vi "Xbox Controller.vi"   [LabVIEW 2011]
uses:
  _GlobalVariables&Libraries/ATV Program Global Variables.vi
types:
  T1 = cluster{"X axis":i32, "Y axis":i32, "Z axis":i32, "X axis rotation":i32, "Y axis rotation":i32, "Z axis rotation":i32, "U axis":i32, "V axis":i32}
  T2 = cluster{"button 1":bool, "button 2":bool, "button 3":bool, "button 4":bool, "button 5":bool, "button 6":bool, "button 7":bool, "button 8":bool, "button 9":bool, "button 10":bool, "button 11":bool, "button 12":bool, "button 13":bool, "button 14":bool, "button 15":bool, "button 16":bool, "button 17":bool, "button 18":bool, "button 19":bool, "button 20":bool, "button 21":bool, "button 22":bool, "button 23":bool, "button 24":bool, "button 25":bool, "button 26":bool, "button 27":bool, "button 28":bool, "button 29":bool, "button 30":bool, "button 31":bool, "button 32":bool}
  T3 = cluster{"pov 1":i32, "pov 2":i32, "pov 3":i32, "pov 4":i32}
  T4 = cluster{"End ATV Program":bool, "E-Stop":bool, "Save Logfile":bool, "Logfile Iteration Delay (ms)":u32, "Loop iteration time (ms)":u32, "Logfile Location":path, "Default GPS Navigation Path":path, "Computer":string, "Default GPS Boundary Path":path}
  T5 = cluster{"Drive Value Output String":string, "Steer Value Output String":string, "Button A":bool, "Button B":bool, "Error Out":errorcluster, "Disable XBox Drive & Steer":bool, "Disable XBox Controller":bool, "XBOX Button Trigger Time (ms)":u32, "Button X":bool, "Button Y":bool}
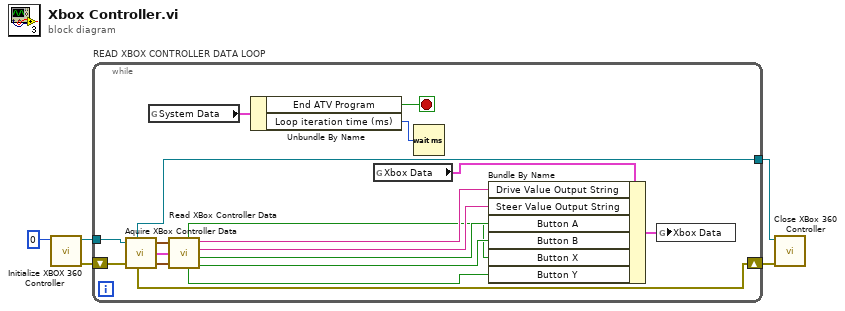
[diagram p0: block diagram]
diagram:
  n1 = call "Initialize XBOX 360 Controller.vi"("XBox Device Index"=0) -> ("Rrror Out"=w3:errorcluster, "Device ID"=w5:refnum<k1>)  [unwired: 8 in, 1 out]
  n2 = while "READ XBOX CONTROLLER DATA LOOP" {
    tunnel: [w20] -> w2
    tunnel: w5 -> [w19]
    shift-right: [w17] -> w1
    shift-left: w3 -> [w18]
    stop <- w9 stop-if-true
    n3 = call "Aquire XBox Controller Data.vi"("Device ID In"=w19, "Error In"=w18) -> ("Device ID Out"=w20:refnum<k1>, "Error Out"=w17:errorcluster, "Axis Info"=w23:T1, "Button Info"=w22:T2, "Direction Info"=w21:T3)  [unwired: 1 in]
    n4 = global read "ATV Program Global Variables.vi" "System Data"() -> (w10:T4)
    n5 = call "Read XBox Controller Data.vi"("Direction Info"=w21, "Button Info"=w22, "Axis Info"=w23) -> ("B"=w12:bool, "Y"=w6:bool, "A"=w13:bool, "Steer Value Output String"=w14:string, "X"=w7:bool, "Drive Value Output String"=w15:string)
    n6 = Unbundle By Name(w10) -> ("End ATV Program"=w9:bool, "Loop iteration time (ms)"=w8:u32)
    n7 = global read "ATV Program Global Variables.vi" "Xbox Data"() -> (w11:T5)
    n8 = Wait (ms)(milliseconds to wait=w8) -> ()  [unwired: 1 out]
    n9 = Bundle By Name(cluster=w11, "Drive Value Output String"=w15, "Steer Value Output String"=w14, "Button A"=w13, "Button B"=w12, "Button X"=w7, "Button Y"=w6) -> (w16:T5)
    n10 = global write "ATV Program Global Variables.vi" "Xbox Data"(w16) -> ()
  }
  n11 = call "Close XBox 360 Controller.vi"("Rrror In"=w1, "Device ID In"=w2) -> ()  [unwired: 9 in, 1 out]
